vi "Read String Register.vi"(7 "PDU Address String Params":T1 items=["Fluid name"=33160, "Capacity unit"=33272, "User tag"=61744], 8 "error in":errorcluster, 11 "MB_TCP session in":refnum<class "MB_Master_TCP.lvclass">) -> (0 "error out":errorcluster, 2 "Value":string, 3 "MB session out":refnum<class "MB_Master_TCP.lvclass">)   [LabVIEW 2024, in "Bronkhorst Flexi-Flow ModbusTCP API.lvlib"]
uses:
  Bronkhorst Flexi-Flow ModbusTCP API.lvlib
  <vilib>/Plasmionique/MB Master/MB_Master_TCP/MB_Master_TCP.lvclass
  C:/Program Files/National Instruments/LabVIEW 2025/vi.lib/Plasmionique/MB Master/MB_Master/MB_Master.lvclass
  PDU Address String Params--ring.ctl
  <vilib>/Plasmionique/MB Master/MB Master.lvlib
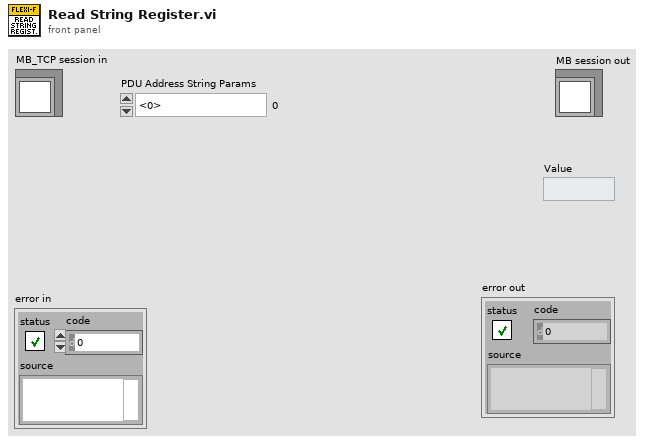
[diagram p1: front panel]
types:
  T1 = typedef "Bronkhorst Flexi-Flow ModbusTCP API.lvlib/PDU Address String Params--ring.ctl" = u16
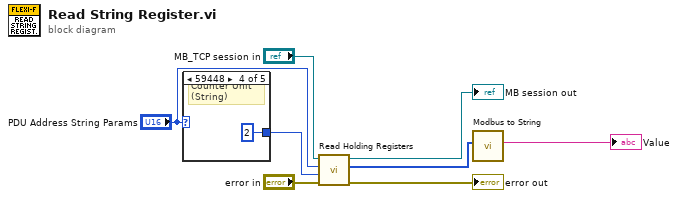
[diagram p0: block diagram]
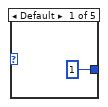
[diagram p2: hidden frame]
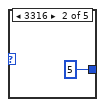
[diagram p3: hidden frame]
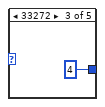
[diagram p4: hidden frame]
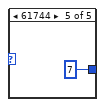
[diagram p5: hidden frame]
diagram:
  n1 = case shown="59448" "PDU Address String Params" {
    tunnel: [u16 1 ("quantity") u16 5 ("quantity") u16 4 ("quantity") u16 2 ("quantity") u16 7 ("quantity")] -> w2
    frame Default {
    }
    frame 3316 {
    }
    frame 33272 {
    }
    frame 59448 {
      # "Counter Unit (String)"
    }
    frame 61744 {
    }
  }
  n2 = call <vilib>:"Read Holding Registers.vi"("error in (no error)"="error in", "quantity"=w2, "starting address"="PDU Address String Params", "MB session in"="MB_TCP session in") -> ("error out"=→"error out":errorcluster, "Registers"=w4:u16[], "MB session out"=→"MB session out":refnum<class "MB_Master_TCP.lvclass">)  [unwired: 5 in]
  n3 = call "Modbus to String.vi"("Registers"=w4) -> ("String"=→"Value":string)  [unwired: 10 in]
